vi "libssh2_knownhost_get - with previous - returns next host.vi"() -> ()   [LabVIEW 2013, in "libssh2_tests.lvlib"]
uses:
  libssh2_tests.lvlib
  libssh2/Known Host Refnum.ctl
  libssh2/libssh2_init_default.vi
  <vilib>/addons/_JKI Toolkits/Caraya/classes/Assert/Assert Equal Value_Variant.vi
  <vilib>/addons/_JKI Toolkits/Caraya/classes/Test/Test.lvclass
  libssh2/libssh2.lvlib
  <vilib>/addons/_JKI Toolkits/Caraya/classes/Assert/Assert.lvclass
panel:
  out "error out":errorcluster
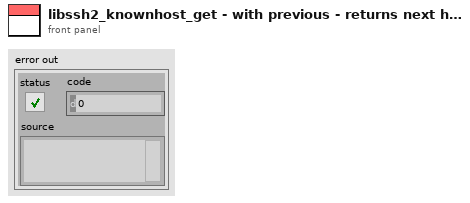
[diagram p1: front panel]
types:
  T1 = typedef "libssh2.lvlib/Known Host Refnum.ctl" = refnum<k1>
  T2 = typedef "libssh2.lvlib/Session Refnum.ctl" = refnum<k1>
  T3 = typedef "libssh2.lvlib/Known Host Collection Refnum.ctl" = refnum<k1>
  T4 = typedef "libssh2.lvlib/libssh2_knownhost.ctl" = cluster{"magic":u32, "node":u64, "name":string, "key":string, "typemask":i32}
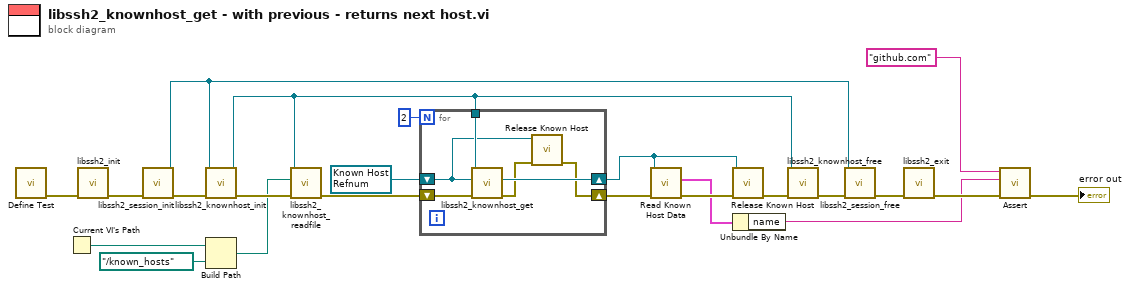
[diagram p0: block diagram]
diagram:
  w2 = T1 refnum items=["Host"] ("next")
  n1 = call <vilib>:"Define Test.vi"() -> ("error out"=w22:errorcluster)  [unwired: 10 in, 1 out]
  n2 = Current VI's Path() -> (path=w13:path)
  n3 = call-poly "libssh2_init.vi"("error in (no error)"=w22) -> ("error out"=w21:errorcluster)  [unwired: 10 in]
  n4 = call "libssh2_session_init.vi"("error in (no error)"=w21) -> ("error out"=w20:errorcluster, "session"=w17:T2)  [unwired: 9 in]
  n5 = call "libssh2_knownhost_init.vi"("error in (no error)"=w20, "session"=w17) -> ("error out"=w15:errorcluster, "known hosts collection"=w10:T3)  [unwired: 8 in]
  n6 = Build Path(base path=w13, name or relative path=path "../known_hosts" ("filename")) -> (appended path=w11:path)
  n7 = call "libssh2_knownhost_readfile.vi"("error in (no error)"=w15, "filename"=w11, "known hosts collection"=w10) -> ("error out"=w14:errorcluster)  [unwired: 7 in, 1 out]
  n8 = for {
    N: 2 -> [_]
    tunnel: w10 -> [w29]
    shift-right: [w28] -> w6
    shift-left: w2 -> [w26]
    shift-right: [w24] -> w8
    shift-left: w14 -> [w27]
    n9 = call "libssh2_knownhost_get.vi"("error in (no error)"=w27, "previous"=w26, "known hosts collection"=w29) -> ("error out"=w25:errorcluster, "next"=w28:T1)  [unwired: 6 in, 1 out]
    n10 = call "Release Known Host.vi"("error in (no error)"=w25, "known host"=w26) -> ("error out"=w24:errorcluster)  [unwired: 9 in]
  }
  n11 = call "Read Known Host Data.vi"("error in (no error)"=w8, "known host"=w6) -> ("error out"=w7:errorcluster, "known host data"=w5:T4)  [unwired: 8 in]
  n12 = call "Release Known Host.vi"("error in (no error)"=w7, "known host"=w6) -> ("error out"=w9:errorcluster)  [unwired: 9 in]
  n13 = Unbundle By Name(w5) -> ("name"=w4:string)
  n14 = call "libssh2_knownhost_free.vi"("error in (no error)"=w9, "known hosts collection"=w10) -> ("error out"=w16:errorcluster)  [unwired: 9 in]
  n15 = call "libssh2_session_free.vi"("error in (no error)"=w16, "session"=w17) -> ("error out"=w19:errorcluster)  [unwired: 9 in]
  n16 = call "libssh2_exit.vi"("error in (no error)"=w19) -> ("error out"=w18:errorcluster)  [unwired: 10 in]
  n17 = call-poly <vilib>:"Assert.vi"("error in (no error)"=w18, "Y"=w4, "X"="github.com" ("key")) -> ("error out"=→"error out":errorcluster)  [unwired: 7 in, 1 out]
